vi "获取昨天到今天任意时间时间段.vi"(9 "当前时间":string, 10 "前一天时间":string) -> (1 "结束时间":string, 2 "开始时间":string)   [LabVIEW 2014]
panel:
  in  "日期格式":string="/"
  out "日":string
  out "月":string
  out "年":string
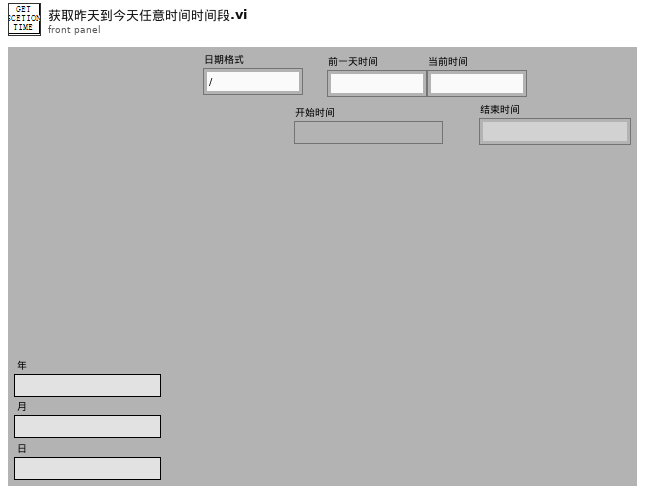
[diagram p1: front panel]
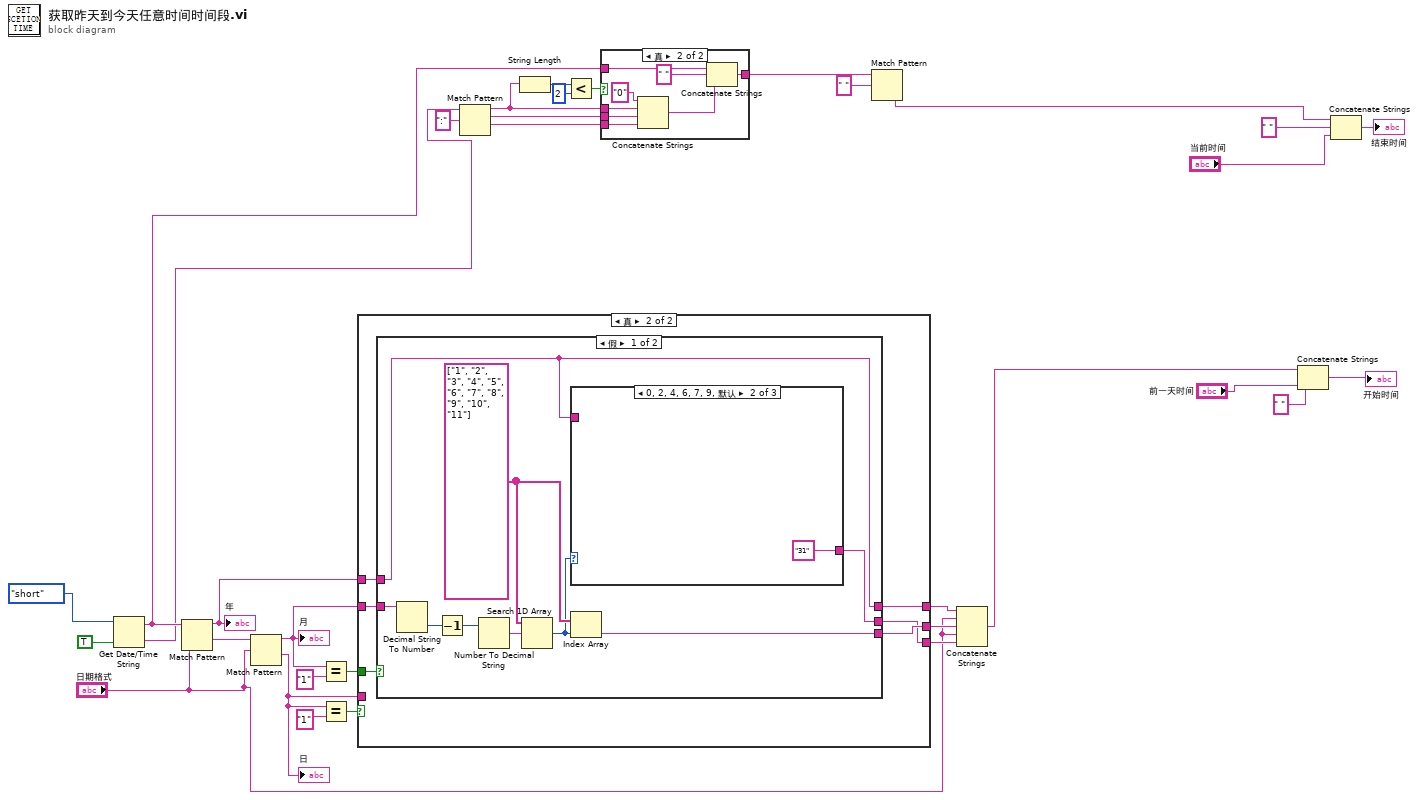
[diagram p0: block diagram]
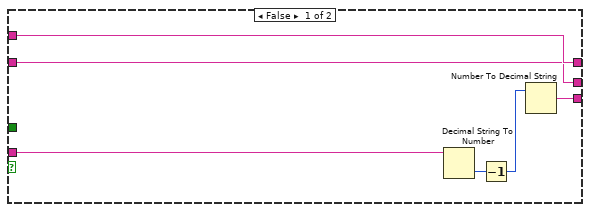
[diagram p2: hidden frame]
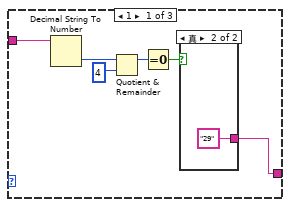
[diagram p3: hidden frame]
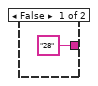
[diagram p4: hidden frame]
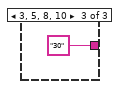
[diagram p5: hidden frame]
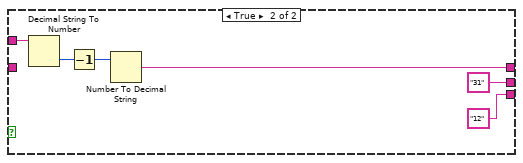
[diagram p6: hidden frame]
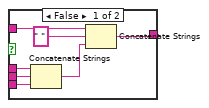
[diagram p7: hidden frame]
diagram:
  n1 = Get Date/Time String(date format (0)=enum16{"short", "long", "abbreviated"}."short" ("日期格式(0)"), want seconds? (F)=TRUE ("需要秒？(F)")) -> (date string=w3:string, time string=w2:string)  [unwired: 1 in]
  n2 = Match Pattern(string=w3, regular expression="日期格式") -> (before substring=w10:string, after substring=w15:string)  [unwired: 1 in, 2 out]
  "年" <- w10
  n3 = Match Pattern(string=w15, regular expression="日期格式") -> (before substring=w6:string, after substring=w5:string)  [unwired: 1 in, 2 out]
  "月" <- w6
  "日" <- w5
  n4 = Equal?(x=w6, y="1") -> (x = y?=w11:bool)
  n5 = Equal?(x=w5, y="1") -> (x = y?=w12:bool)
  n6 = case shown="真" w12 {
    tunnel: w11 -> [_ w45]
    tunnel: w10 -> [w35 w44]
    tunnel: [w35 w43] -> w9
    tunnel: [w34 w42] -> w8
    tunnel: [w36 w41] -> w7
    tunnel: w6 -> [w34 w40]
    tunnel: w5 -> [w37 _]
    frame False {
      n7 = Decimal String To Number(string=w37) -> (number=w39:i32)  [unwired: 2 in, 1 out]
      n8 = Decrement(x=w39) -> (x-1=w38:i32)
      n9 = Number To Decimal String(number=w38) -> (decimal integer string=w36:string)  [unwired: 1 in]
    }
    frame True {
      n10 = case shown="假" w45 {
        tunnel: w44 -> [w50 w69]
        tunnel: [w50 w67] -> w43
        tunnel: [w51 "12" ("正则表达式")] -> w42
        tunnel: [w54 "31" ("正则表达式")] -> w41
        tunnel: w40 -> [w47 _]
        frame False {
          w53 = string[] ["1", "2", "3", "4", "5", "6", "7", "8", "9", "10", "11"] ("一维数组")
          n11 = Decimal String To Number(string=w47) -> (number=w48:i32)  [unwired: 2 in, 1 out]
          n12 = Decrement(x=w48) -> (x-1=w49:i32)
          n13 = Number To Decimal String(number=w49) -> (decimal integer string=w46:string)  [unwired: 1 in]
          n14 = Search 1D Array(1D array=w53, element=w46) -> (index of element=w52:i32)  [unwired: 1 in]
          n15 = case shown="0, 2, 4, 6, 7, 9, 默认" w52 {
            tunnel: [w55 "31" "30"] -> w54
            tunnel: w50 -> [w56 _ _]
            frame 1 {
              n16 = Decimal String To Number(string=w56) -> (number=w57:i32)  [unwired: 2 in, 1 out]
              n17 = Quotient & Remainder(x=w57, y=4) -> (x-y*floor(x/y)=w59:i32)  [unwired: 1 out]
              n18 = Equal To 0?(x=w59) -> (x = 0?=w60:bool)
              n19 = case shown="真" w60 {
                tunnel: ["28" "29"] -> w55
                frame False {
                }
                frame True {
                }
              }
            }
            frame 0, 2, 4, 6, 7, 9, Default {
            }
            frame 3, 5, 8, 10 {
            }
          }
          n20 = Index Array(array=w53, index=w52) -> (element=w51:string)
        }
        frame True {
          n21 = Decimal String To Number(string=w69) -> (number=w68:i32)  [unwired: 2 in, 1 out]
          n22 = Decrement(x=w68) -> (x-1=w70:i32)
          n23 = Number To Decimal String(number=w70) -> (decimal integer string=w67:string)  [unwired: 1 in]
        }
      }
    }
  }
  n24 = Match Pattern(string=w2, regular expression=":" ("正则表达式")) -> (before substring=w27:string, match substring=w28:string, after substring=w29:string)  [unwired: 1 in, 1 out]
  n25 = String Length(string=w27) -> (length=w24:i32)
  n26 = Less?(x=w24, y=2) -> (x < y?=w26:bool)
  n27 = case shown="真" w26 {
    tunnel: w27 -> [w75 w82]
    tunnel: w3 -> [w74 w85]
    tunnel: w28 -> [w72 w81]
    tunnel: w29 -> [w71 w80]
    tunnel: [w73 w78] -> w22
    frame False {
      n28 = Concatenate Strings(w75, w72, w71) -> (w76:string)
      n29 = Concatenate Strings(w74, " " ("字符串"), w76) -> (w73:string)
    }
    frame True {
      n30 = Concatenate Strings("0" ("字符串"), w82, w81, w80) -> (w79:string)
      n31 = Concatenate Strings(w85, " " ("字符串"), w79) -> (w78:string)
    }
  }
  n32 = Match Pattern(string=w22, regular expression=" " ("字符串")) -> (before substring=w33:string)  [unwired: 1 in, 3 out]
  n33 = Concatenate Strings(w9, "日期格式", w8, "日期格式", w7) -> (w4:string)
  n34 = Concatenate Strings(w4, " " ("字符串"), "前一天时间") -> (→"开始时间":string)
  n35 = Concatenate Strings(w33, " " ("字符串"), "当前时间") -> (→"结束时间":string)
